vi "oa_IIR Preprocess Filter with Multi-channel Signals.vi"(6 "reset":bool, 8 "error in (no error)":errorcluster, 9 "IIR Filter Cluster":T1, 10 "signals in":waveform(dbl)[](array[waveform]), 11 "filter history in":cluster{"shift register type":dbl[]}[](array[cluster])) -> (0 "error out":errorcluster, 2 "signals out":waveform(dbl)[](array[waveform]), 3 "filter history out":cluster{"shift register type":dbl[]}[](array[cluster]))   [LabVIEW 2017, in "SoundVib_RefDataProcess.lvlib"]
uses:
  <vilib>/addons/Sound and Vibration/Order Analysis/Referece Data Processing/SoundVib_RefDataProcess.lvlib
  <vilib>/Analysis/NI_AALBase.lvlib
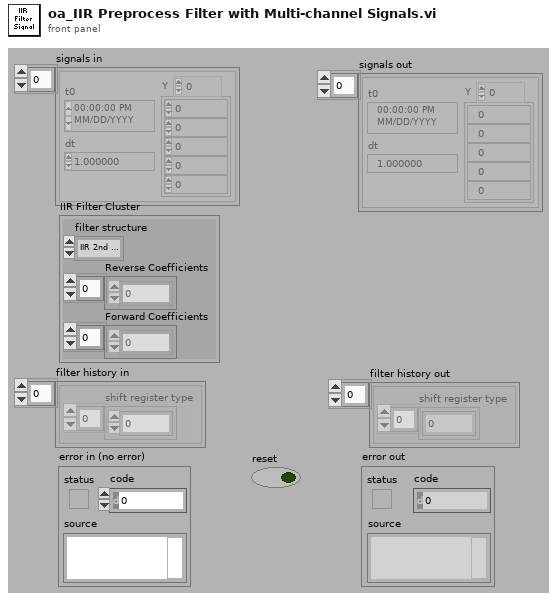
[diagram p1: front panel]
types:
  T1 = cluster{"filter structure":enum32{"IIR 2nd Order", "IIR 4th Order"}, "Reverse Coefficients":dbl[], "Forward Coefficients":dbl[]}
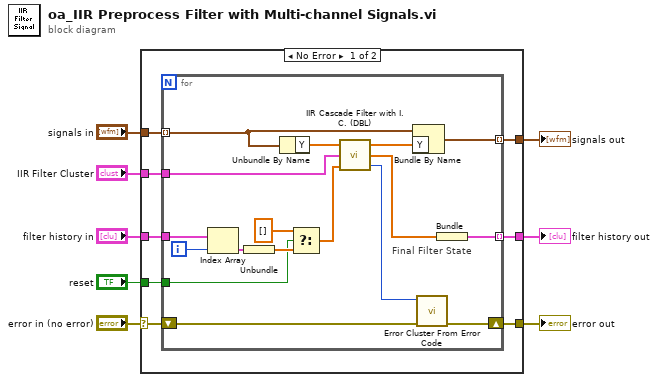
[diagram p0: block diagram]
diagram:
  n1 = case shown="No Error" "error in (no error)" {
    selector: "error in (no error)" -> [w9 w35]
    tunnel: "signals in" -> [w16 w34]
    tunnel: [w15 w34] -> w7
    tunnel: "IIR Filter Cluster" -> [w14 _]
    tunnel: "filter history in" -> [w13 _]
    tunnel: "reset" -> [w12 _]
    tunnel: [w11 _] -> w2
    tunnel: [w10 w35] -> w1
    frame No Error {
      n2 = for {
        tunnel: w14 -> [w24]
        tunnel: [w28] -> w11 mode=indexing
        tunnel: w13 -> [w30]
        tunnel: w16 -> [w27] mode=indexing
        tunnel: [w33] -> w15 mode=indexing
        shift-right: [w31] -> w10
        shift-left: w9 -> [w32]
        tunnel: w12 -> [w20]
        i -> [w29]
        # "Final Filter State"
        n3 = Index Array(array=w30, index=w29) -> (element=w23:cluster{"shift register type":dbl[]})
        n4 = Unbundle(w23) -> ("shift register type"=w21:dbl[])
        n5 = Unbundle By Name(w27) -> ("Y"=w26:dbl[])
        n6 = Select(t=dbl[] [] ("shift register type"), s=w20, f=w21) -> (s? t:f=w19:dbl[])
        n7 = call <vilib>:"IIR Cascade Filter with I.C. (DBL).vi"("Initial Filter State"=w19, "IIR Filter Cluster"=w24, "X"=w26) -> ("error"=w17:i32, "Final Filter State"=w18:dbl[], "Filtered X"=w25:dbl[])
        n8 = Bundle By Name(cluster=w27, "Y"=w25) -> (w33:waveform(dbl))
        n9 = call <vilib>:"Error Cluster From Error Code.vi"("error in (no error)"=w32, "error code (0)"=w17) -> ("error out"=w31:errorcluster)  [unwired: 7 in]
        n10 = Bundle("Final Filter State"=w18) -> (w28:cluster{"Final Filter State":dbl[]})  [unwired: 1 in]
      }
    }
    frame Error {
    }
  }
  "signals out" <- w7
  "error out" <- w1
  "filter history out" <- w2
